vi "Move_relative_Peregrine.vi"(5 "Address":u8, 7 "Relative move distance":i32, 8 "error":errorcluster, 9 "Speed input":i16, 10 "Acceleration input":u16, 11 "Handle in":refnum<visa-resource-name>) -> (0 "error out":errorcluster, 1 "New target":i32, 2 "Current position":i32, 3 "Handle out":refnum<visa-resource-name>)   [LabVIEW 2019]
panel:
  out "Query speed":i16
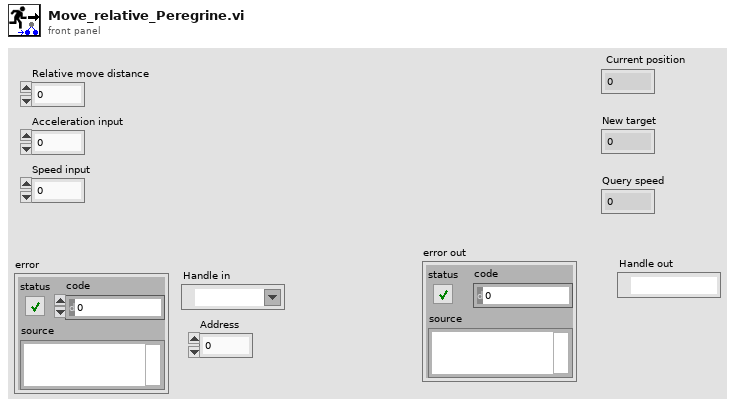
[diagram p1: front panel]
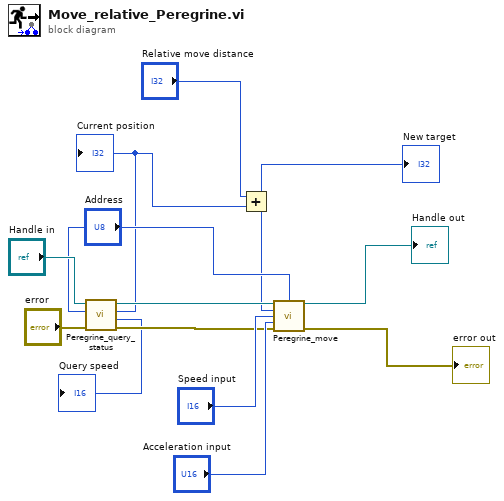
[diagram p0: block diagram]
diagram:
  n1 = call "Peregrine_query_status.vi"("error"="error", "Address"="Address", "Handle in"="Handle in") -> ("error out"=w7:errorcluster, "Speed"=→"Query speed":i16, "Position"=w2:i32, "Handle out"=w8:refnum<visa-resource-name>)  [unwired: 4 in, 1 out]
  "Current position" <- w2
  n2 = Add(x="Relative move distance", y=w2) -> (x+y=w1:i32)
  "New target" <- w1
  n3 = call "Peregrine_move.vi"("Handle in"=w8, "Address"="Address", "Target"=w1, "Speed"="Speed input", "Acceleration"="Acceleration input", "error"=w7) -> ("Handle out"=→"Handle out":refnum<visa-resource-name>, "error out"=→"error out":errorcluster)  [unwired: 8 in]
